vi "ConvertParametersToJSON.vi"(11 "Parameters":T1) -> (3 "JSON string":string)   [LabVIEW 2020]
uses:
  Parameters.ctl
  CGrapherDGML.lvclass
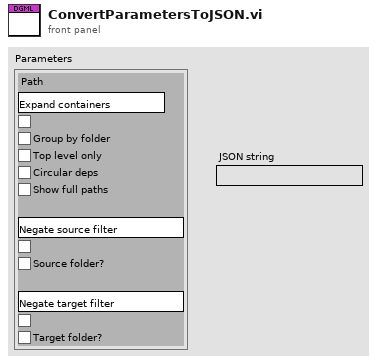
[diagram p1: front panel]
types:
  T1 = typedef "DefaultExtensions.lvlib/CGrapherDGML.lvclass/Parameters.ctl" = cluster{"Path":string, "Expand containers":bool, "Group by folder":bool, "Top level only":bool, "Circular deps":bool, "Show full paths":bool, "Source filter":string, "Negate source filter":bool, "Source folder?":bool, "Target filter":string, "Negate target filter":bool, "Target folder?":bool}
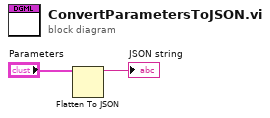
[diagram p0: block diagram]
diagram:
  n1 = Flatten To JSON(anything="Parameters") -> (JSON string=→"JSON string":string)  [unwired: 2 in, 1 out]
